vi "Execute.vi"(8 "error in (no error)":errorcluster, 9 "Workspace":T1, 10 "Control In":T2, 11 "Secure Syringe in":refnum<class "SecureRelease Syringe.lvclass">) -> (0 "error out":errorcluster, 2 "Control Out":T2, 3 "Secure Syringe out":refnum<class "SecureRelease Syringe.lvclass">)   [LabVIEW 2020, in "SecureRelease Syringe.lvclass"]
uses:
  SecureRelease Syringe.lvclass
  Controller/Controllers.ctl
  Controller/I-O/I-O.lvclass
  Controller/Dispenser/Dispenser.lvclass
  C:/Program Files (x86)/Aerotech/A3200/LabVIEW/2010/Bin/Aerotech.A3200.dll
  Program Files (x86)/Aerotech/A3200/LabVIEW/2010/Bin/Aerotech.A3200.dll
  Workspace/Workspace.ctl
  SecureRelease Syringe.lvclass/SecureRelease Syringe.ctl
  Controller/Motion/A3200/A3200.lvclass
  Dispense/Dispense.lvclass
  Controller/Controller.lvclass
  Workspace/Fixture.lvclass
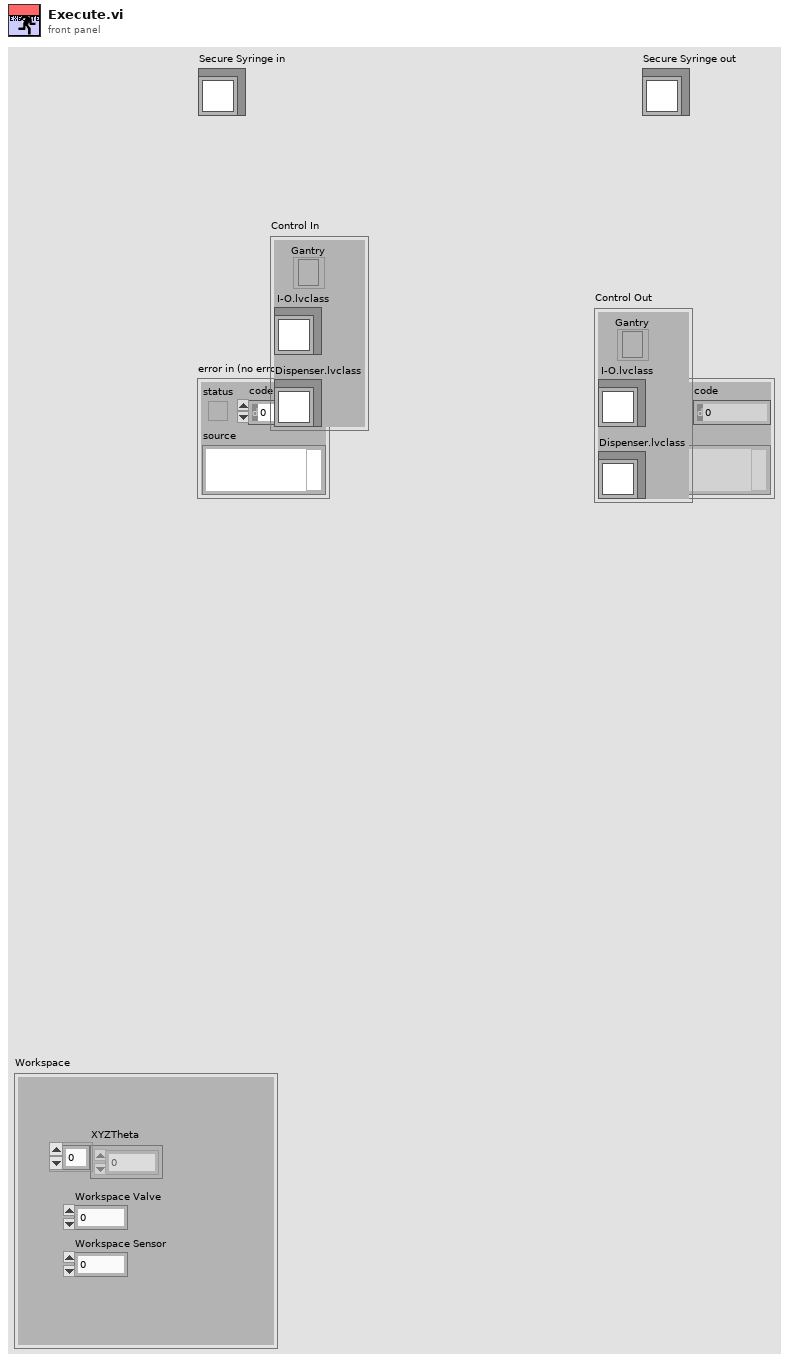
[diagram p1: front panel]
types:
  T1 = typedef "Fixture.lvclass/Workspace.ctl" = cluster{"XYZTheta":dbl[], "Workspace Valve":i32, "Workspace Sensor":i32}
  T2 = typedef "Controller.lvclass/Controllers.ctl" = cluster{"I-O.lvclass":refnum<class "I-O.lvclass">, "Dispenser.lvclass":refnum<class "Dispenser.lvclass">, "Gantry":refnum<k24>}
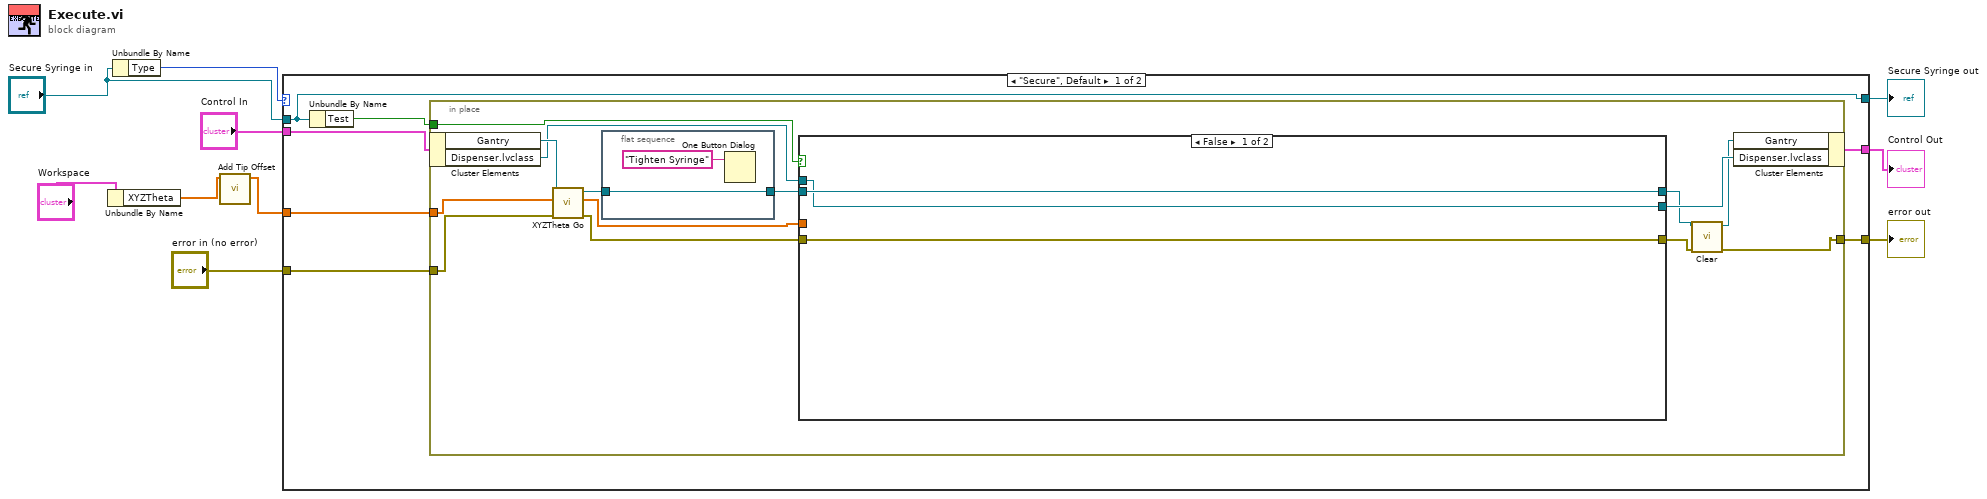
[diagram p0: block diagram]
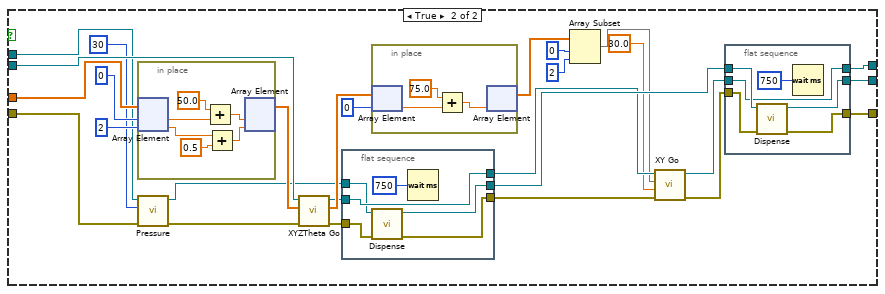
[diagram p2: hidden frame]
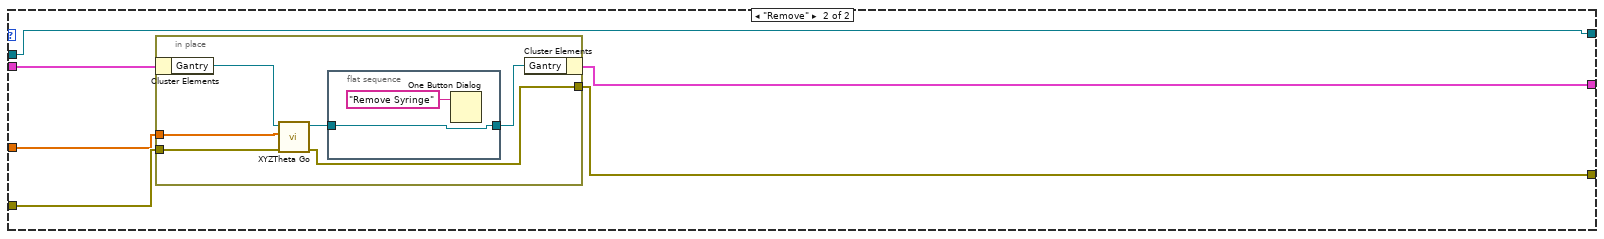
[diagram p3: hidden frame]
diagram:
  n1 = Unbundle By Name("Workspace") -> ("XYZTheta"=w1:dbl[])
  n2 = Unbundle By Name("Secure Syringe in") -> ("Type"=w6:enum16{"Secure", "Remove"})
  n3 = call "Add Tip Offset.vi"("XYZTheta"=w1) -> ("XYZTheta"=w2:dbl[])  [unwired: 10 in]
  n4 = case shown="\"Secure\", Default" w6 {
    tunnel: "Secure Syringe in" -> [w14 w88]
    tunnel: [w14 w88] -> w10
    tunnel: "Control In" -> [w17 w89]
    tunnel: [w16 w90] -> w8
    tunnel: "error in (no error)" -> [w13 w87]
    tunnel: [w12 w86] -> w4
    tunnel: w2 -> [w11 w85]
    frame "Secure", Default {
      n5 = Unbundle By Name(w14) -> ("Test"=w15:bool)
      n6 = in-place {
        in-place-border: w15 -> [w27]
        in-place-border: w13 -> [w24]
        in-place-border: [w18] -> w12
        in-place-border: w11 -> [w22]
        n7 = in-place-cluster #1(w17) -> ("Gantry"=w31:refnum<k24>, "Dispenser.lvclass"=w26:refnum<class "Dispenser.lvclass">)
        n8 = call "XYZTheta Go.vi"("error in (no error)"=w24, "XYZTheta In"=w22, "Gantry In"=w31) -> ("error out"=w23:errorcluster, "XYZTheta Out"=w28:dbl[], "Gantry Out"=w30:refnum<k24>)  [unwired: 6 in]
        n9 = flat-sequence {
          tunnel: [w83] -> w29
          tunnel: w30 -> [w83]
          frame #0 {
            n10 = One Button Dialog(message="Tighten Syringe") -> ()  [unwired: 1 in, 1 out]
          }
        }
        n11 = case shown="False" w27 {
          tunnel: w29 -> [w34 w61]
          tunnel: [w34 w50] -> w20
          tunnel: w28 -> [_ w60]
          tunnel: w26 -> [w33 w54]
          tunnel: [w33 w48] -> w25
          tunnel: w23 -> [w32 w40]
          tunnel: [w32 w35] -> w19
          frame False {
          }
          frame True {
            n12 = in-place {
              n13 = in-place-array #2(w60, 0, 2) -> (w82:dbl, w80:dbl)
              n14 = Add(x=50.0, y=w82) -> (x+y=w77:dbl)
              n15 = Add(x=w80, y=0.5) -> (x+y=w78:dbl)
              n16 = in-place-array #2(w77, w78) -> (w57:dbl[])  [unwired: 2 out]
            }
            n17 = call-dynamic "Pressure.vi"("error in (no error)"=w40, "Pressure"=i16 30, "Dispenser in"=w54) -> ("error out"=w39:errorcluster, "Dispenser out"=w51:refnum<class "Dispenser.lvclass">)  [unwired: 7 in]
            n18 = call "XYZTheta Go.vi"("error in (no error)"=w39, "XYZTheta In"=w57, "Gantry In"=w61) -> ("error out"=w38:errorcluster, "XYZTheta Out"=w56:dbl[], "Gantry Out"=w52:refnum<k24>)  [unwired: 6 in]
            n19 = flat-sequence {
              tunnel: [w73] -> w44
              tunnel: w52 -> [w73]
              tunnel: w51 -> [w72]
              tunnel: [w70] -> w49
              tunnel: w38 -> [w69]
              tunnel: [w68] -> w37
              frame #0 {
                n20 = call-dynamic "Dispense.vi"("error in (no error)"=w69, "Dispenser in"=w72) -> ("error out"=w68:errorcluster, "Dispenser out"=w70:refnum<class "Dispenser.lvclass">)  [unwired: 8 in]
                n21 = Wait (ms)(milliseconds to wait=u32 750) -> ()  [unwired: 1 out]
              }
            }
            n22 = in-place {
              n23 = in-place-array #3(w56, 0) -> (w76:dbl)
              n24 = Add(x=75.0, y=w76) -> (x+y=w74:dbl)
              n25 = in-place-array #3(w74) -> (w47:dbl[])  [unwired: 1 out]
            }
            n26 = Array Subset(array=w47, index=0, length=2) -> (w42:dbl[])
            n27 = call "XY Go.vi"("error in (no error)"=w37, "Speed"=30.0, "XY"=w42, "Gantry In"=w44) -> ("error out"=w36:errorcluster, "Gantry Out"=w43:refnum<k24>)  [unwired: 6 in]
            n28 = flat-sequence {
              tunnel: [w64] -> w50
              tunnel: w49 -> [w67]
              tunnel: [w65] -> w48
              tunnel: w43 -> [w64]
              tunnel: w36 -> [w63]
              tunnel: [w62] -> w35
              frame #0 {
                n29 = call-dynamic "Dispense.vi"("error in (no error)"=w63, "Dispenser in"=w67) -> ("error out"=w62:errorcluster, "Dispenser out"=w65:refnum<class "Dispenser.lvclass">)  [unwired: 8 in]
                n30 = Wait (ms)(milliseconds to wait=u32 750) -> ()  [unwired: 1 out]
              }
            }
          }
        }
        n31 = call "Clear.vi"("error in (no error)"=w19, "Gantry In"=w20) -> ("error out"=w18:errorcluster, "Gantry Out"=w21:refnum<k24>)  [unwired: 8 in]
        n32 = in-place-cluster #1("Gantry"=w21, "Dispenser.lvclass"=w25) -> (w16:T2)
      }
    }
    frame "Remove" {
      n33 = in-place {
        in-place-border: w85 -> [w93]
        in-place-border: w87 -> [w92]
        in-place-border: [w91] -> w86
        n34 = in-place-cluster #4(w89) -> ("Gantry"=w96:refnum<k24>)
        n35 = call "XYZTheta Go.vi"("error in (no error)"=w92, "XYZTheta In"=w93, "Gantry In"=w96) -> ("error out"=w91:errorcluster, "Gantry Out"=w95:refnum<k24>)  [unwired: 6 in, 1 out]
        n36 = flat-sequence {
          tunnel: w95 -> [w98]
          tunnel: [w98] -> w94
          frame #0 {
            n37 = One Button Dialog(message="Remove Syringe") -> ()  [unwired: 1 in, 1 out]
          }
        }
        n38 = in-place-cluster #4("Gantry"=w94) -> (w90:T2)
      }
    }
  }
  "error out" <- w4
  "Secure Syringe out" <- w10
  "Control Out" <- w8
